vi "Tree_FocusTag_Tests.vi"(11 "error in":errorcluster) -> (15 "error out":errorcluster)   [LabVIEW 2016, in "DronaTest.lvlib"]
uses:
  DronaTest.lvlib
  APIs/Stimulus/ControlValue/SetValueAuto.vi
  APIs/Stimulus/ControlValue/Controls/Tree/SetValueByItemTag.vi
  APIs/Assert/AssertControlValue/Controls/Tree/AssertValueByFocusTag.vi
  <vilib>/addons/_JKI Toolkits/Caraya/classes/Assert/Assert Equal Value_Variant.vi
  <vilib>/addons/_JKI Toolkits/Caraya/classes/Assert/Assert Error.vi
  <vilib>/addons/_JKI Toolkits/Caraya/classes/Test/Test.lvclass
  Drona.lvlib
  <vilib>/SLL Toolkit/SLL Debug/SLL Debug.lvlib
  APIs/Stimulus/ControlValue/ControlValue.lvlib
  <vilib>/addons/_JKI Toolkits/Caraya/classes/Assert/Assert.lvclass
  APIs/Stimulus/ControlValue/Controls/Tree/StimulusTree.lvlib
  APIs/Assert/AssertControlValue/Controls/Tree/AssertTree.lvlib
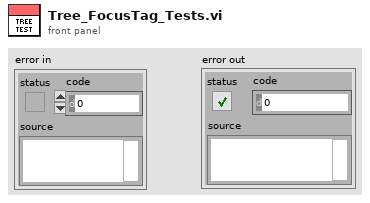
[diagram p1: front panel]
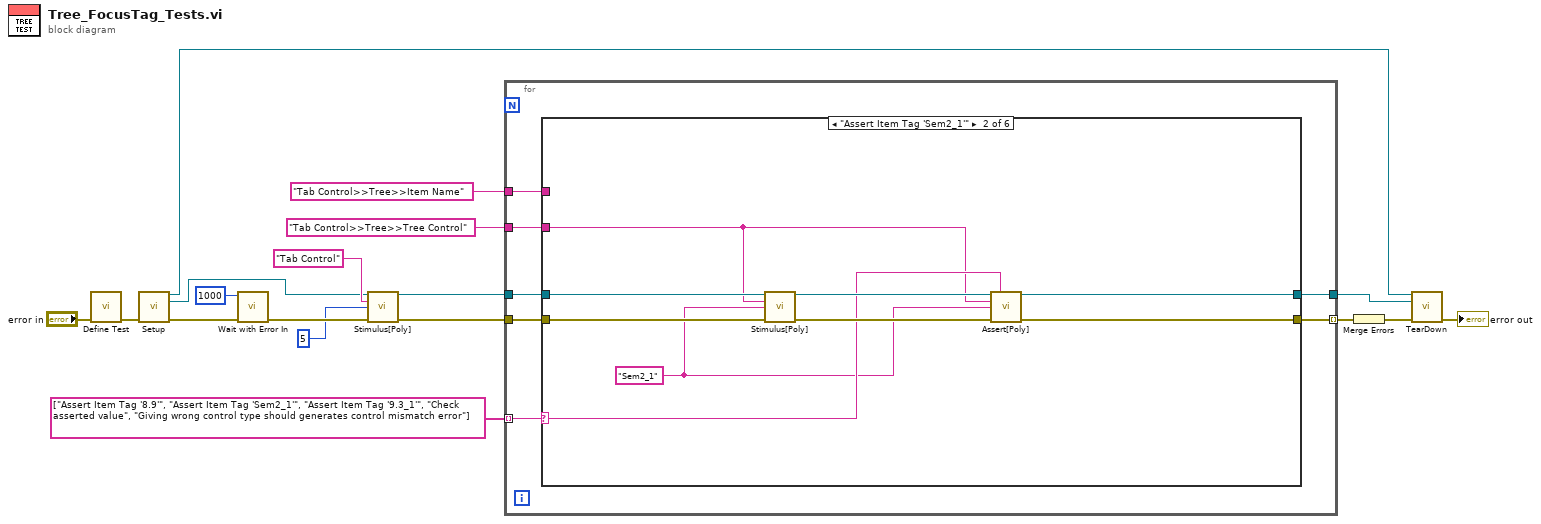
[diagram p0: block diagram]
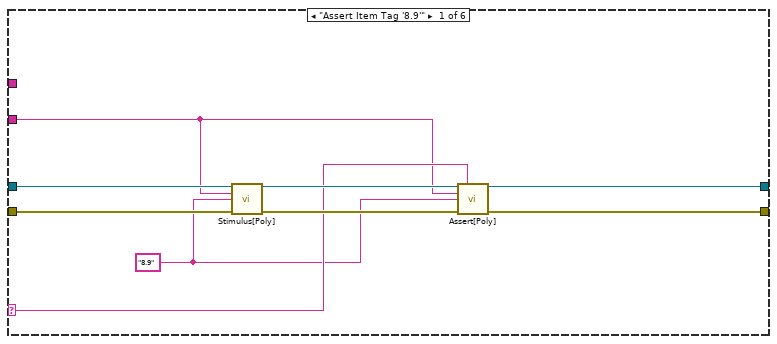
[diagram p2: hidden frame]
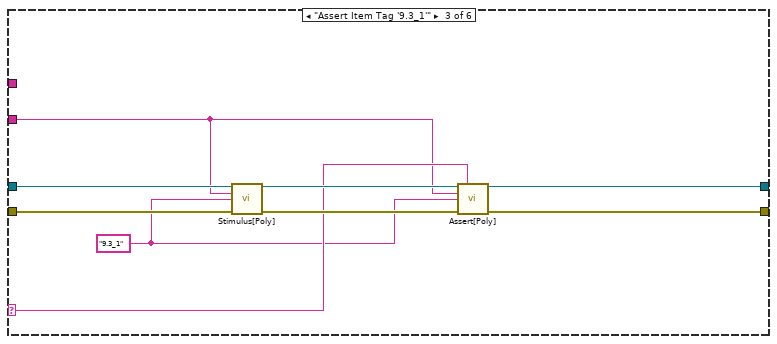
[diagram p3: hidden frame]
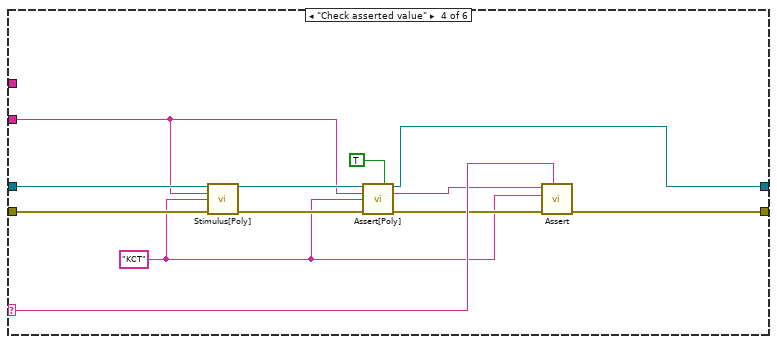
[diagram p4: hidden frame]
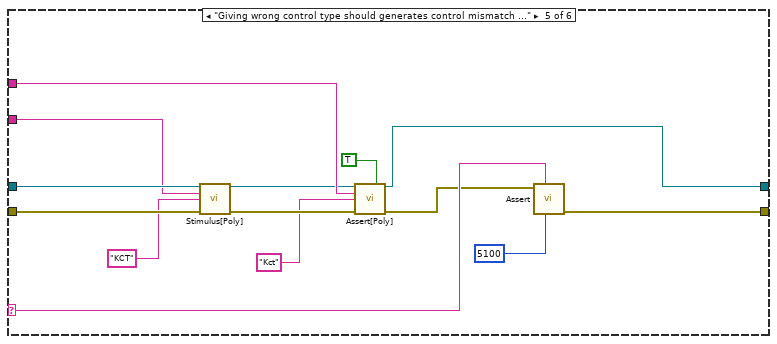
[diagram p5: hidden frame]
diagram:
  n1 = call <vilib>:"Define Test.vi"("error in (no error)"="error in") -> ("error out"=w7:errorcluster)  [unwired: 9 in, 1 out]
  n2 = call "Setup.vi"("error in (no error)"=w7) -> ("Application Ref"=w2:refnum<vi>, "VI out"=w6:refnum<vi>, "error out"=w5:errorcluster)  [unwired: 12 in]
  n3 = call <vilib>:"Wait with Error In.vi"("error in (no error)"=w5, "milliseconds to wait"=u32 1000) -> ("error out"=w16:errorcluster)  [unwired: 9 in]
  n4 = call-poly "Stimulus[Poly].vi"("VI Reference In"=w6, "Control Path"="Tab Control", "Value (Signaling)"=5, "error in"=w16) -> ("VI Reference Out"=w12:refnum<vi>, "error out"=w15:errorcluster)  [unwired: 10 in]
  n5 = for {
    tunnel: w12 -> [w24]
    tunnel: "Tab Control>>Tree>>Tree Control" ("Control Path") -> [w23]
    tunnel: "Tab Control>>Tree>>Item Name" ("Control Path") -> [w22]
    tunnel: string[] ["Assert Item Tag '8.9'", "Assert Item Tag 'Sem2_1'", "Assert Item Tag '9.3_1'", "Check asserted value", "Giving wrong control type should generates control mismatch error"] -> [w20] mode=indexing
    tunnel: [w19] -> w3
    tunnel: w15 -> [w25]
    tunnel: [w21] -> w8 mode=indexing
    n6 = case shown="\"Assert Item Tag 'Sem2_1'\"" w20 {
      selector: w20 -> [w28 w37 w46 w61 w75 _]
      tunnel: w25 -> [w34 w43 w52 w64 w78 w80]
      tunnel: w24 -> [w33 w42 w51 w63 w77 w79]
      tunnel: w23 -> [w26 w35 w45 w57 w73 _]
      tunnel: w22 -> [_ _ _ _ w71 _]
      tunnel: [w30 w39 w48 w62 w76 w80] -> w21
      tunnel: [w29 w38 w47 w58 w68 w79] -> w19
      frame "Assert Item Tag '8.9'" {
        w27 = "8.9" ("Item Name")
        n7 = call-poly "Stimulus[Poly].vi"("VI Reference In"=w33, "Control Path"=w26, "Item Tag"=w27, "Error In"=w34) -> ("VI Reference Out"=w31:refnum<vi>, "Error Out"=w32:errorcluster)  [unwired: 10 in]
        n8 = call-poly "Assert[Poly].vi"("VI Reference In"=w31, "Test Label"=w28, "Control Path"=w26, "Focus Item Tag"=w27, "Error In"=w32) -> ("VI Reference Out"=w29:refnum<vi>, "Error Out"=w30:errorcluster)  [unwired: 8 in, 1 out]
      }
      frame "Assert Item Tag 'Sem2_1'" {
        w36 = "Sem2_1" ("Item Name")
        n9 = call-poly "Stimulus[Poly].vi"("VI Reference In"=w42, "Control Path"=w35, "Item Tag"=w36, "Error In"=w43) -> ("VI Reference Out"=w40:refnum<vi>, "Error Out"=w41:errorcluster)  [unwired: 10 in]
        n10 = call-poly "Assert[Poly].vi"("VI Reference In"=w40, "Test Label"=w37, "Control Path"=w35, "Focus Item Tag"=w36, "Error In"=w41) -> ("VI Reference Out"=w38:refnum<vi>, "Error Out"=w39:errorcluster)  [unwired: 8 in, 1 out]
      }
      frame "Assert Item Tag '9.3_1'" {
        w44 = "9.3_1" ("Item Name")
        n11 = call-poly "Stimulus[Poly].vi"("VI Reference In"=w51, "Control Path"=w45, "Item Tag"=w44, "Error In"=w52) -> ("VI Reference Out"=w49:refnum<vi>, "Error Out"=w50:errorcluster)  [unwired: 10 in]
        n12 = call-poly "Assert[Poly].vi"("VI Reference In"=w49, "Test Label"=w46, "Control Path"=w45, "Focus Item Tag"=w44, "Error In"=w50) -> ("VI Reference Out"=w47:refnum<vi>, "Error Out"=w48:errorcluster)  [unwired: 8 in, 1 out]
      }
      frame "Check asserted value" {
        w54 = "KCT" ("Item Name")
        n13 = call-poly "Stimulus[Poly].vi"("VI Reference In"=w63, "Control Path"=w57, "Item Tag"=w54, "Error In"=w64) -> ("VI Reference Out"=w59:refnum<vi>, "Error Out"=w60:errorcluster)  [unwired: 10 in]
        n14 = call-poly "Assert[Poly].vi"("VI Reference In"=w59, "Assert Only? (F)"=TRUE, "Control Path"=w57, "Focus Item Tag"=w54, "Error In"=w60) -> ("VI Reference Out"=w58:refnum<vi>, "Asserted Value"=w55:string, "Error Out"=w56:errorcluster)  [unwired: 8 in]
        n15 = call-poly <vilib>:"Assert.vi"("Label"=w61, "error in (no error)"=w56, "Y"=w54, "X"=w55) -> ("error out"=w62:errorcluster)  [unwired: 6 in, 1 out]
      }
      frame "Giving wrong control type should generates control mismatch error" {
        n16 = call-poly "Stimulus[Poly].vi"("VI Reference In"=w77, "Control Path"=w73, "Item Tag"="KCT" ("Item Name"), "Error In"=w78) -> ("VI Reference Out"=w69:refnum<vi>, "Error Out"=w72:errorcluster)  [unwired: 10 in]
        n17 = call-poly "Assert[Poly].vi"("VI Reference In"=w69, "Assert Only? (F)"=TRUE, "Control Path"=w71, "Focus Item Tag"="Kct" ("Item Name"), "Error In"=w72) -> ("VI Reference Out"=w68:refnum<vi>, "Error Out"=w67:errorcluster)  [unwired: 8 in, 1 out]
        n18 = call-poly <vilib>:"Assert.vi"("error code (1)"=5100, "Label"=w75, "Error?"=w67) -> ("error out"=w76:errorcluster)  [unwired: 7 in, 1 out]
      }
      frame Default {
      }
    }
  }
  n19 = Merge Errors(w8) -> (w4:errorcluster)
  n20 = call "TearDown.vi"("Application Ref"=w2, "VI in"=w3, "error in (no error)"=w4) -> ("error out"=→"error out":errorcluster)  [unwired: 12 in]
